vi "Send_String_Short.vi"(8 "error in (no error)":errorcluster, 10 "String":string, 11 "SpinCoater in":refnum<class "SpinCoater.lvclass">) -> (0 "error out":errorcluster, 3 "SpinCoater out":refnum<class "SpinCoater.lvclass">)   [LabVIEW 2020, in "SpinCoater.lvclass"]
uses:
  <instrlib>/Classes/SpinCoater/SpinCoater.lvclass
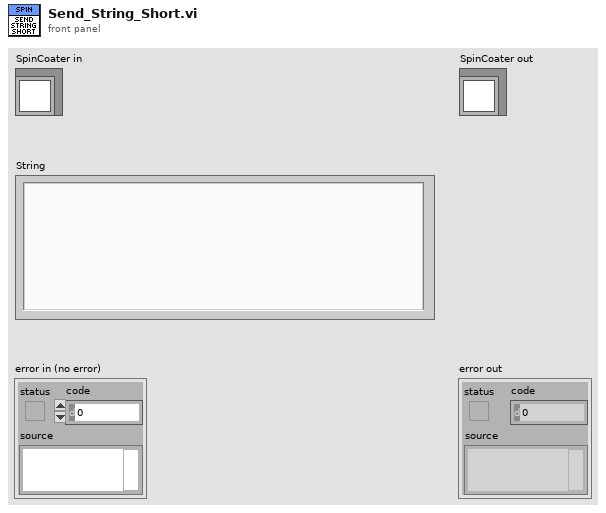
[diagram p1: front panel]
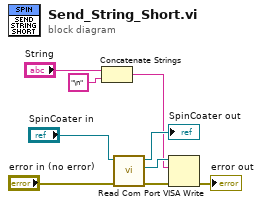
[diagram p0: block diagram]
diagram:
  n1 = Concatenate Strings("String", "\n") -> (w1:string)
  n2 = call-dynamic "Read Com Port.vi"("error in (no error)"="error in (no error)", "SpinCoater in"="SpinCoater in") -> ("error out"=w5:errorcluster, "Com Port"=w4:refnum<visa-resource-name>, "SpinCoater out"=→"SpinCoater out":refnum<class "SpinCoater.lvclass">)  [unwired: 7 in]
  n3 = VISA Write(VISA resource name=w4, write buffer=w1, error in (no error)=w5) -> (error out=→"error out":errorcluster)  [unwired: 2 out]
